vi "EditOptions.vi"(8 "error in":errorcluster, 11 "group in":refnum<class "_Group.lvclass">) -> (0 "error out":errorcluster, 1 "edit options":T1, 2 "subnodes class":T2, 3 "group out":refnum<class "_Group.lvclass">)   [LabVIEW 2013, in "_Group.lvclass"]
doc: "This VI Contains the options for the Menu that will be displayed when doing right click on an item\nThe subnodes class configures which nodes can be added to this nodes\nAnd the edit options determine which options are available for the node.\n\nThis configuration is stored in this VI in case some dynamic configuration is required for the menu options or subnodes.\n\nAll VIs must overide this method"
uses:
  _Group.lvclass
  CEF_TreeControl/Node/SubNodeCluster.ctl
  CEF_TreeControl/Node/NodeMenuOptions.ctl
  CEF_TreeControl/Node/NISE_CEF_Node.lvclass
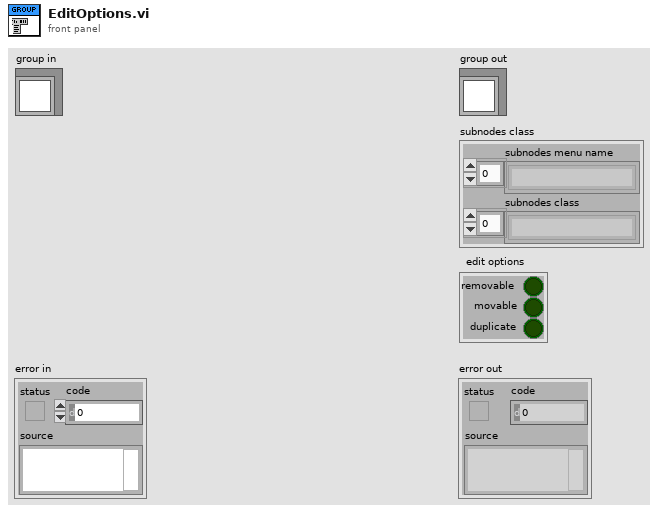
[diagram p1: front panel]
types:
  T1 = typedef "NISE_CEF_Node.lvclass/NodeMenuOptions.ctl" = cluster{"removable":bool, "movable":bool, "duplicate":bool}
  T2 = typedef "NISE_CEF_Node.lvclass/SubNodeCluster.ctl" = cluster{"subnodes menu name":string[], "subnodes class":string[]}
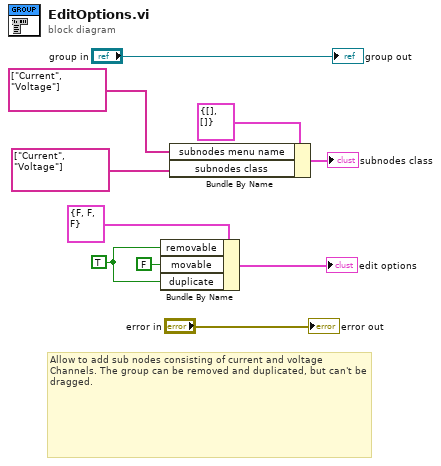
[diagram p0: block diagram]
diagram:
  w7 = TRUE ("movable")
  # "Allow to add sub nodes consisting of current and voltage Channels. The group can be removed and duplicated, but can't be dragged."
  n1 = Bundle By Name(cluster=T1 {"removable"=FALSE, "movable"=FALSE, "duplicate"=FALSE} ("edit options 2"), "removable"=w7, "movable"=FALSE, "duplicate"=w7) -> (→"edit options":T1)
  n2 = Bundle By Name(cluster=T2 {"subnodes menu name"=[], "subnodes class"=[]} ("subnodes class"), "subnodes menu name"=string[] ["Current", "Voltage"] ("subnodes class"), "subnodes class"=string[] ["Current", "Voltage"]) -> (→"subnodes class":T2)
  "error out" <- "error in"
  "group out" <- "group in"
